vi "LibXML_CreateNewXMLFile.vi"(6 "Assign this Schema":bool, 8 "error in":errorcluster, 9 "Schema-Cluster":T1, 10 "Root element name":string, 11 "file path":path) -> (0 "error out":errorcluster, 2 "new doc out":u32, 3 "new file path":path=path "D:/bhs/programming/XML-toolkit/personnel.xml")   [LabVIEW 2019, in "Tools.lvlib" / "LibXML.lvlib"]
doc: "Creates a new XML-file with root-element name and without any subtags"
uses:
  LibXML.lvlib
panel:
  # "This software is FREE licensed under the GNU Lesser General Public License (see license.txt).."
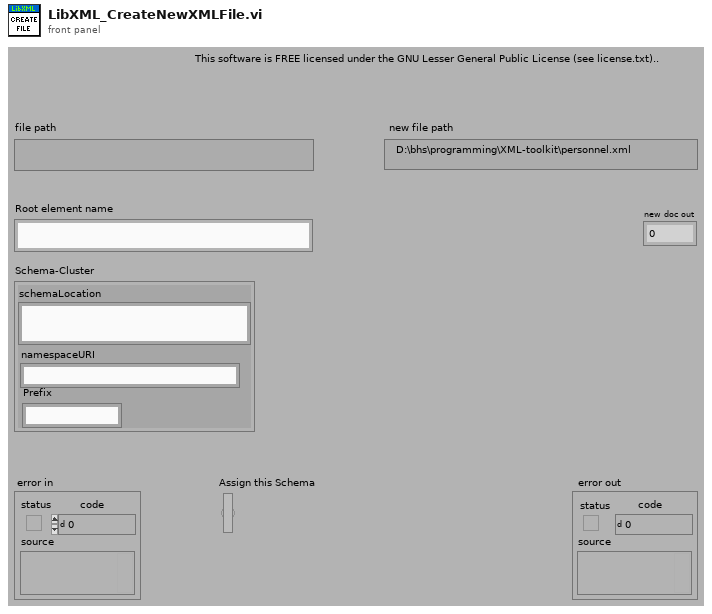
[diagram p1: front panel]
types:
  T1 = cluster{"schemaLocation":string, "namespaceURI":string, "Prefix":string}
  T2 = enum16{"open", "open or create", "create or replace", "create", "open (read only)"}
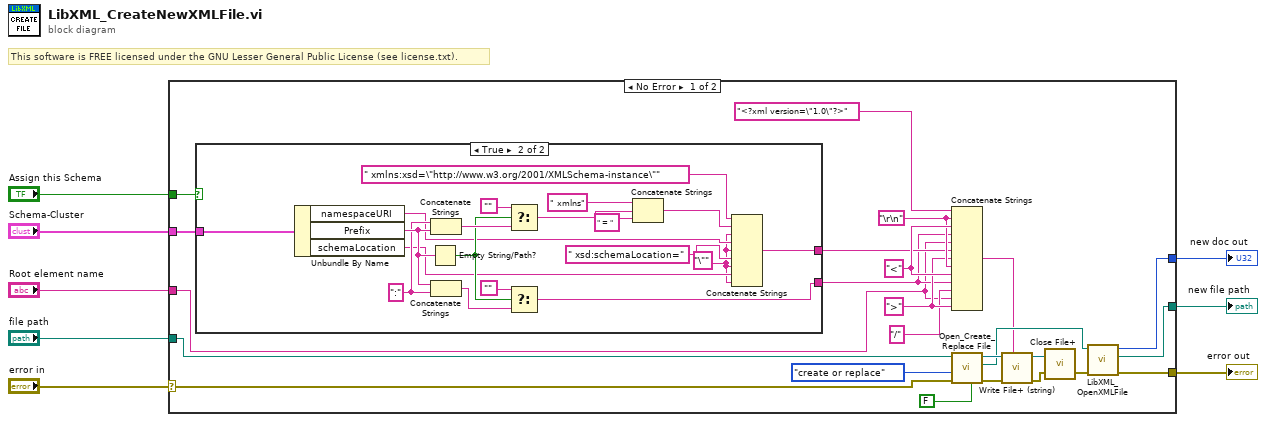
[diagram p0: block diagram]
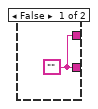
[diagram p2: hidden frame]
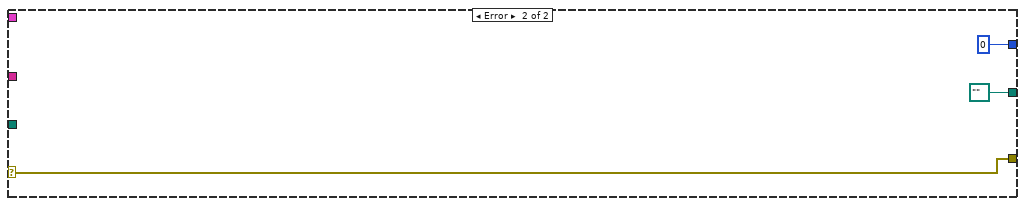
[diagram p3: hidden frame]
diagram:
  # "This software is FREE licensed under the GNU Lesser General Public License (see license.txt)."
  n1 = case shown="No Error" "error in" {
    selector: "error in" -> [w10 w53]
    tunnel: [w32 w53] -> w8
    tunnel: [w31 path "" ("new file path")] -> w7
    tunnel: [w30 u32 0 ("doc")] -> w6
    tunnel: "Assign this Schema" -> [w22 _]
    tunnel: "Schema-Cluster" -> [w21 _]
    tunnel: "Root element name" -> [w20 _]
    tunnel: "file path" -> [w13 _]
    frame No Error {
      w26 = ">"
      w28 = "<"
      w27 = "\r\n"
      n2 = case shown="True" w22 {
        tunnel: [w33 w39] -> w25
        tunnel: [w33 w40] -> w24
        tunnel: w21 -> [_ w34]
        frame False {
          w33 = ""
        }
        frame True {
          w44 = ":"
          w35 = "\""
          n3 = Unbundle By Name(w34) -> ("namespaceURI"=w38:string, "Prefix"=w45:string, "schemaLocation"=w36:string)
          n4 = Empty String/Path?(string/path=w45) -> (empty?=w42:bool)
          n5 = Concatenate Strings(w44, w45) -> (w51:string)
          n6 = Concatenate Strings(w45, w44) -> (w43:string)
          n7 = Select(t="", s=w42, f=w51) -> (s? t:f=w50:string)
          n8 = Select(t="", s=w42, f=w43) -> (s? t:f=w40:string)
          n9 = Concatenate Strings(" xmlns", w50, " = ") -> (w48:string)
          n10 = Concatenate Strings(" xmlns:xsd=\"http://www.w3.org/2001/XMLSchema-instance\"", w48, w35, w38, w35, " xsd:schemaLocation=", w35, w36, w35) -> (w39:string)
        }
      }
      n11 = Concatenate Strings("<?xml version=\"1.0\"?>", w27, w28, w24, w20, w25, w26, w27, w28, w24, "/", w20, w26) -> (w12:string)
      n12 = call <vilib>:"Open_Create_Replace File.vi"("advisory dialog? (display:T)"=FALSE, "error in (no error)"=w10, "function (open:0)"=T2."create or replace", "file path"=w13) -> ("error out"=w19:errorcluster, "new file path"=w15:path, "refnum"=w16:refnum<file>)  [unwired: 4 in, 1 out]
      n13 = call <vilib>:"Write File+ (string).vi"("string"=w12, "error in (no error)"=w19, "refnum"=w16) -> ("error out"=w18:errorcluster, "dup refnum"=w17:refnum<file>)  [unwired: 4 in, 1 out]
      n14 = call <vilib>:"Close File+.vi"("error in (no error)"=w18, "refnum"=w17) -> ("error out"=w11:errorcluster)  [unwired: 3 in, 2 out]
      n15 = call "LibXML_OpenXMLFile.vi"("error in"=w11, "file path"=w15) -> ("error out"=w32:errorcluster, "new file path"=w31:path, "doc"=w30:u32)  [unwired: 7 in]
    }
    frame Error {
    }
  }
  "error out" <- w8
  "new file path" <- w7
  "new doc out" <- w6
